vi "class_data.vi"() -> ()   [LabVIEW 2017, in "GenericComponent.lvclass"]
uses:
  GenericComponent.lvclass
  main/labview_source/type_definitions/clusters/controls_refs.ctl
  main/labview_source/type_definitions/enumerations/run_mode_enum.ctl
  components/Objective/GenericObjective/GenericObjective/GenericObjective.lvclass
  NoteBook/Notebook/Notebook.lvclass
panel:
  in  "loaded components":string[](array[string])
  in  "username":string
  in  "notebook":refnum<class "Notebook.lvclass">
  in  "file name base":string
  in  "data folder path":path
  in  "current objective":refnum<class "GenericObjective.lvclass">
  out "shut down?":bool
  in  "run mode":T1
  in  "config files base folder":path
  out "control references":T2
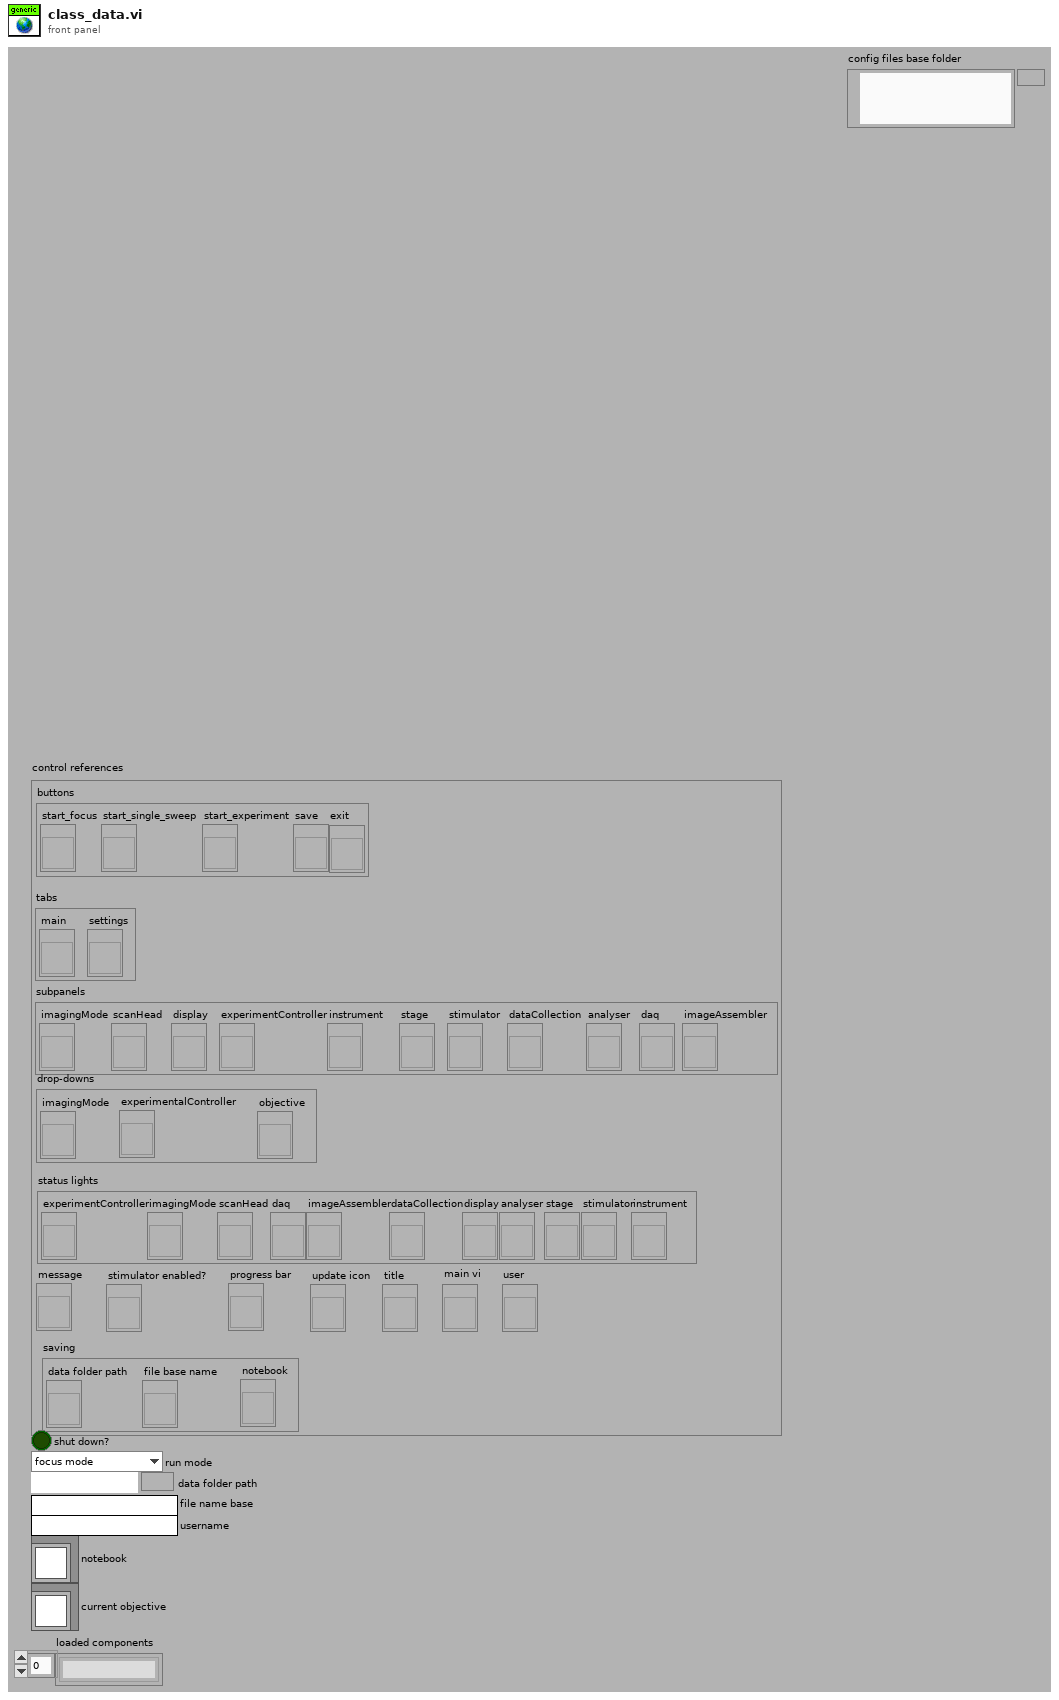
[diagram p1: front panel]
types:
  T1 = typedef "run_mode_enum.ctl" = enum16{"focus mode", "single sweep mode", "experiment mode"}
  T2 = typedef "controls_refs.ctl" = cluster{"buttons":cluster{"start_focus":refnum<vi>, "start_single_sweep":refnum<vi>, "start_experiment":refnum<vi>, "save":refnum<vi>, "exit":refnum<vi>}, "tabs":cluster{"main":refnum<vi>, "settings":refnum<vi>}, "subpanels":cluster{"imagingMode":refnum<vi>, "scanHead":refnum<vi>, "display":refnum<vi>, "experimentController":refnum<vi>, "instrument":refnum<vi>, "stage":refnum<vi>, "stimulator":refnum<vi>, "dataCollection":refnum<vi>, "analyser":refnum<vi>, "daq":refnum<vi>, "imageAssembler":refnum<vi>}, "drop-downs":cluster{"imagingMode":refnum<vi>, "experimentalController":refnum<vi>, "objective":refnum<vi>}, "status lights":cluster{"experimentController":refnum<vi>, "imagingMode":refnum<vi>, "scanHead":refnum<vi>, "daq":refnum<vi>, "imageAssembler":refnum<vi>, "dataCollection":refnum<vi>, "display":refnum<vi>, "analyser":refnum<vi>, "stage":refnum<vi>, "stimulator":refnum<vi>, "instrument":refnum<vi>}, "message":refnum<vi>, "stimulator enabled?":refnum<vi>, "saving":cluster{"data folder path":refnum<vi>, "file base name":refnum<vi>, "notebook":refnum<vi>}, "progress bar":refnum<vi>, "update icon":refnum<vi>, "title":refnum<vi>, "main vi":refnum<vi>, "user":refnum<vi>}
diagram:
